vi "Conversor_mm_a_pasos.vi"(8 "error in (no error)":errorcluster, 9 "pasosZ":dbl, 10 "pasosY":dbl, 11 "pasosX":dbl) -> (0 "error out":errorcluster, 1 "PASOS EN Z":u32, 2 "PASOS EN Y":u32, 3 "PASOS EN X":u32)   [LabVIEW 2019, in "SHARED VI'S.lvlib"]
uses:
  SHARED VI'S.lvlib
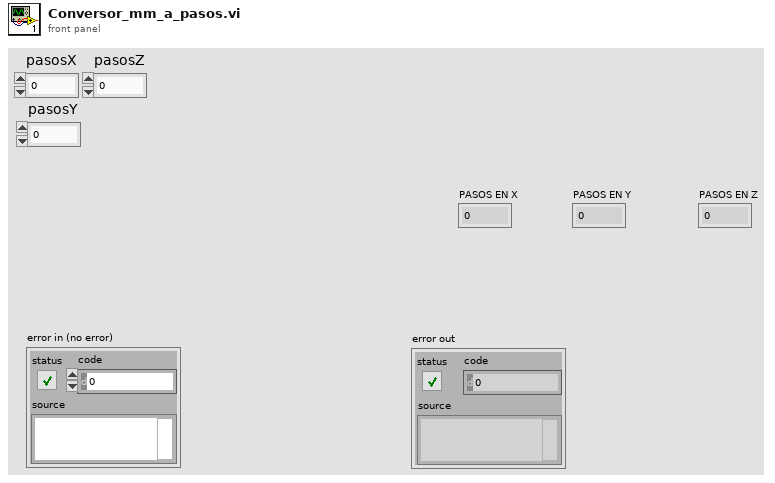
[diagram p1: front panel]
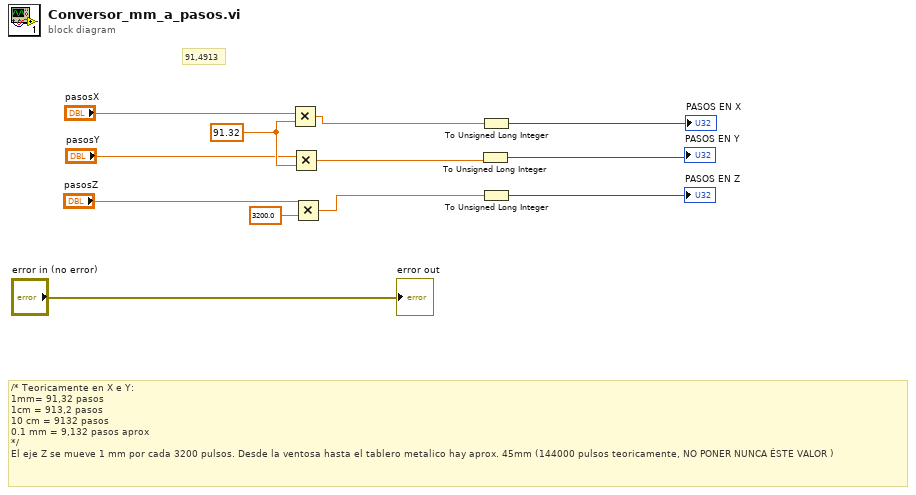
[diagram p0: block diagram]
diagram:
  w12 = 91.32
  # "91,4913"
  # "/* Teoricamente en X e Y:\n1mm= 91,32 pasos\n1cm = 913,2 pasos\n10 cm = 9132 pasos\n0.1 mm = 9,132 pasos aprox\n*/\nEl eje Z se mueve 1 mm por cada 3200 pulsos. Desde la ventosa hasta el tablero metalico hay aprox. 45mm (144000 pulsos teoricamente, NO PONER NUNCA ÉSTE VALOR )"
  n1 = Multiply(x="pasosX", y=w12) -> (x*y=w9:dbl)
  n2 = Multiply(x="pasosY", y=w12) -> (x*y=w8:dbl)
  n3 = Multiply(x="pasosZ", y=3200.0) -> (x*y=w7:dbl)
  n4 = To Unsigned Long Integer(number=w8) -> (unsigned 32bit integer=→"PASOS EN Y":u32)
  n5 = To Unsigned Long Integer(number=w9) -> (unsigned 32bit integer=→"PASOS EN X":u32)
  n6 = To Unsigned Long Integer(number=w7) -> (unsigned 32bit integer=→"PASOS EN Z":u32)
  "error out" <- "error in (no error)"
